vi "Autonomous Independent.vi"() -> ()   [LabVIEW 2012]
doc: "This VI is called when autonomous begins, and will automatically be terminated when autonomous ends. You can carry out timed or sensor driven robot movement independently without needing to return to the caller."
uses:
  <vilib>/Rock Robotics/WPI/Relay/WPI_RelayValue.ctl
  Robot Global Data.vi
  <vilib>/Rock Robotics/WPI/RobotDrive/WPI_RobotDriveGetSetRefNum.vi
  <vilib>/Rock Robotics/WPI/Joystick/WPI_JoystickGetSetRefNum.vi
  <vilib>/Rock Robotics/WPI/RobotDrive/WPI_RobotDriveArcadeDrive_Standard(NoSaturation).vi
panel:
  in  "Array of robot movements 2":T1(array[cluster]) {"Y Joystick Value" scale=1.0..-1.0; "X Joystick Value" scale=-1.0..1.0}
  out "Current Movement, for debugging 2":T2 {"Y Joystick Value" scale=1.0..-1.0; "X Joystick Value" scale=-1.0..1.0}
  out "Current Movement, for debugging":T2 {"Y Joystick Value" scale=1.0..-1.0; "X Joystick Value" scale=-1.0..1.0}
  in  "Array of robot movements":T1(array[cluster]) {"Y Joystick Value" scale=1.0..-1.0; "X Joystick Value" scale=-1.0..1.0}
  # "Be sure to right-click and choose Data Operations>>Make Current Value default if you want to save the array values with the VI"
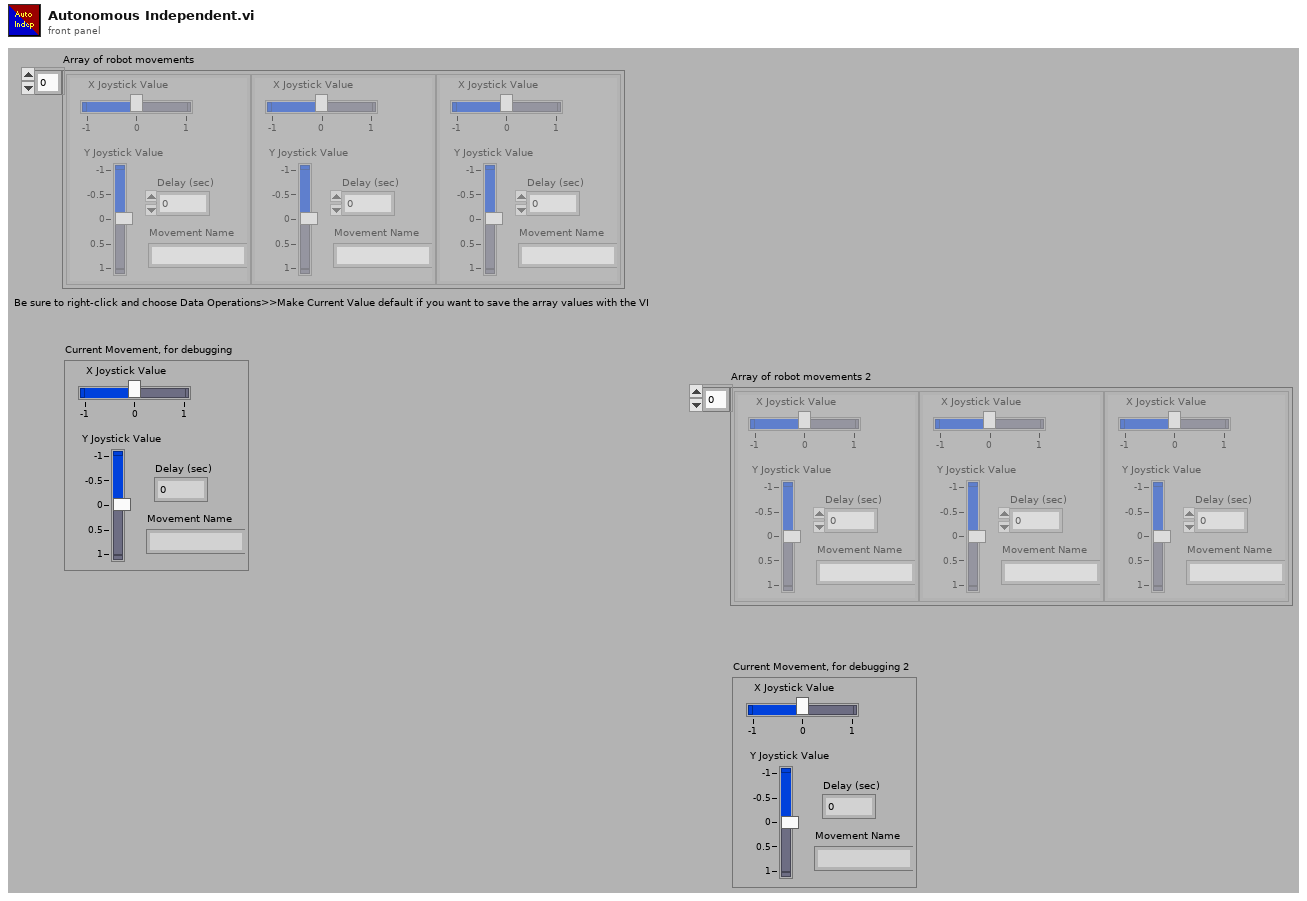
[diagram p1: front panel]
types:
  T1 = cluster{"X Joystick Value":dbl, "Y Joystick Value":dbl, "Delay (sec)":dbl, "Movement Name":string}[]
  T2 = cluster{"X Joystick Value":dbl, "Y Joystick Value":dbl, "Delay (sec)":dbl, "Movement Name":string}
  T3 = typedef "WPI_RelayValue.ctl" = enum16{"Off", "On", "Forward", "Reverse"}
  T4 = typedef "WPI_RobotDriveDevRef.ctl" = cluster{"DevStatus":errorcluster, "Motors[]":T5[], "Square Inputs":bool, "Max Output":dbl, "Isochronous":bool}
  T5 = typedef "WPI_MotorControlDeviceRef.ctl" = cluster{"DeviceStatus":errorcluster, "Type":enum16{"PWM", "CAN"}, "PWM":cluster{"Digital Module":T6, "PWM Channel":T7, "DeadBand":T8}, "CAN":cluster{"Device Number":u8, "Control Mode":T9, "Semaphore":T10, "Max Vout":dbl}, "Invert":bool, "TransformRef":T11, "InvTransformRef":T11}
  T6 = typedef "FPGA_TypedefDigitalModule.ctl" = enum16{"Digital Module 1", "Digital Module 2"}
  T7 = typedef "FPGA_DIOPWMChannel.ctl" = enum8{"PWM 1", "PWM 2", "PWM 3", "PWM 4", "PWM 5", "PWM 6", "PWM 7", "PWM 8", "PWM 9", "PWM 10", "Invalid"}
  T8 = typedef "WPI_PWMDeadband.ctl" = cluster{"Name":string, "maxPositivePwm":i32, "minPositivePwm":i32, "centerPwm":i32, "maxNegativePwm":i32, "minNegativePwm":i32, "angularRange":u16}
  T9 = typedef "WPI_CANJaguar_ControlMode.ctl" = enum8{"Percent VBus", "Current", "Speed", "Position", "Voltage"}
  T10 = typedef "Semaphore RefNum" = refnum<k1>
  T11 = typedef "WPI_PWMTransform_ConPane.ctl" = refnum<vi>
  T12 = typedef "WPI_RelayDevRef.ctl" = cluster{"DevStatus":errorcluster, "Relay Channel":T13, "Digital Module":T6, "Relay Direction":T14}
  T13 = typedef "FPGA_DIORelayChannel.ctl" = enum8{"Relay 1", "Relay 2", "Relay 3", "Relay 4", "Relay 5", "Relay 6", "Relay 7", "Relay 8", "Invalid"}
  T14 = typedef "WPI_RelayDirection.ctl" = enum16{"Both directions", "Forward only", "Reverse only"}
  T15 = typedef "WPI_JoystickDevRef.ctl" = cluster{"Device":T16}
  T16 = typedef "WPI_JoystickDeviceEnum.ctl" = enum16{"USB 1", "USB 2", "USB 3", "USB 4", "Kinect 1", "Kinect 2"}
  T17 = cluster{"axis 1 (x)":dbl, "axis 2 (y)":dbl, "axis 3 (throttle)":dbl, "axis 4":dbl, "axis 5":dbl, "axis 6":dbl}
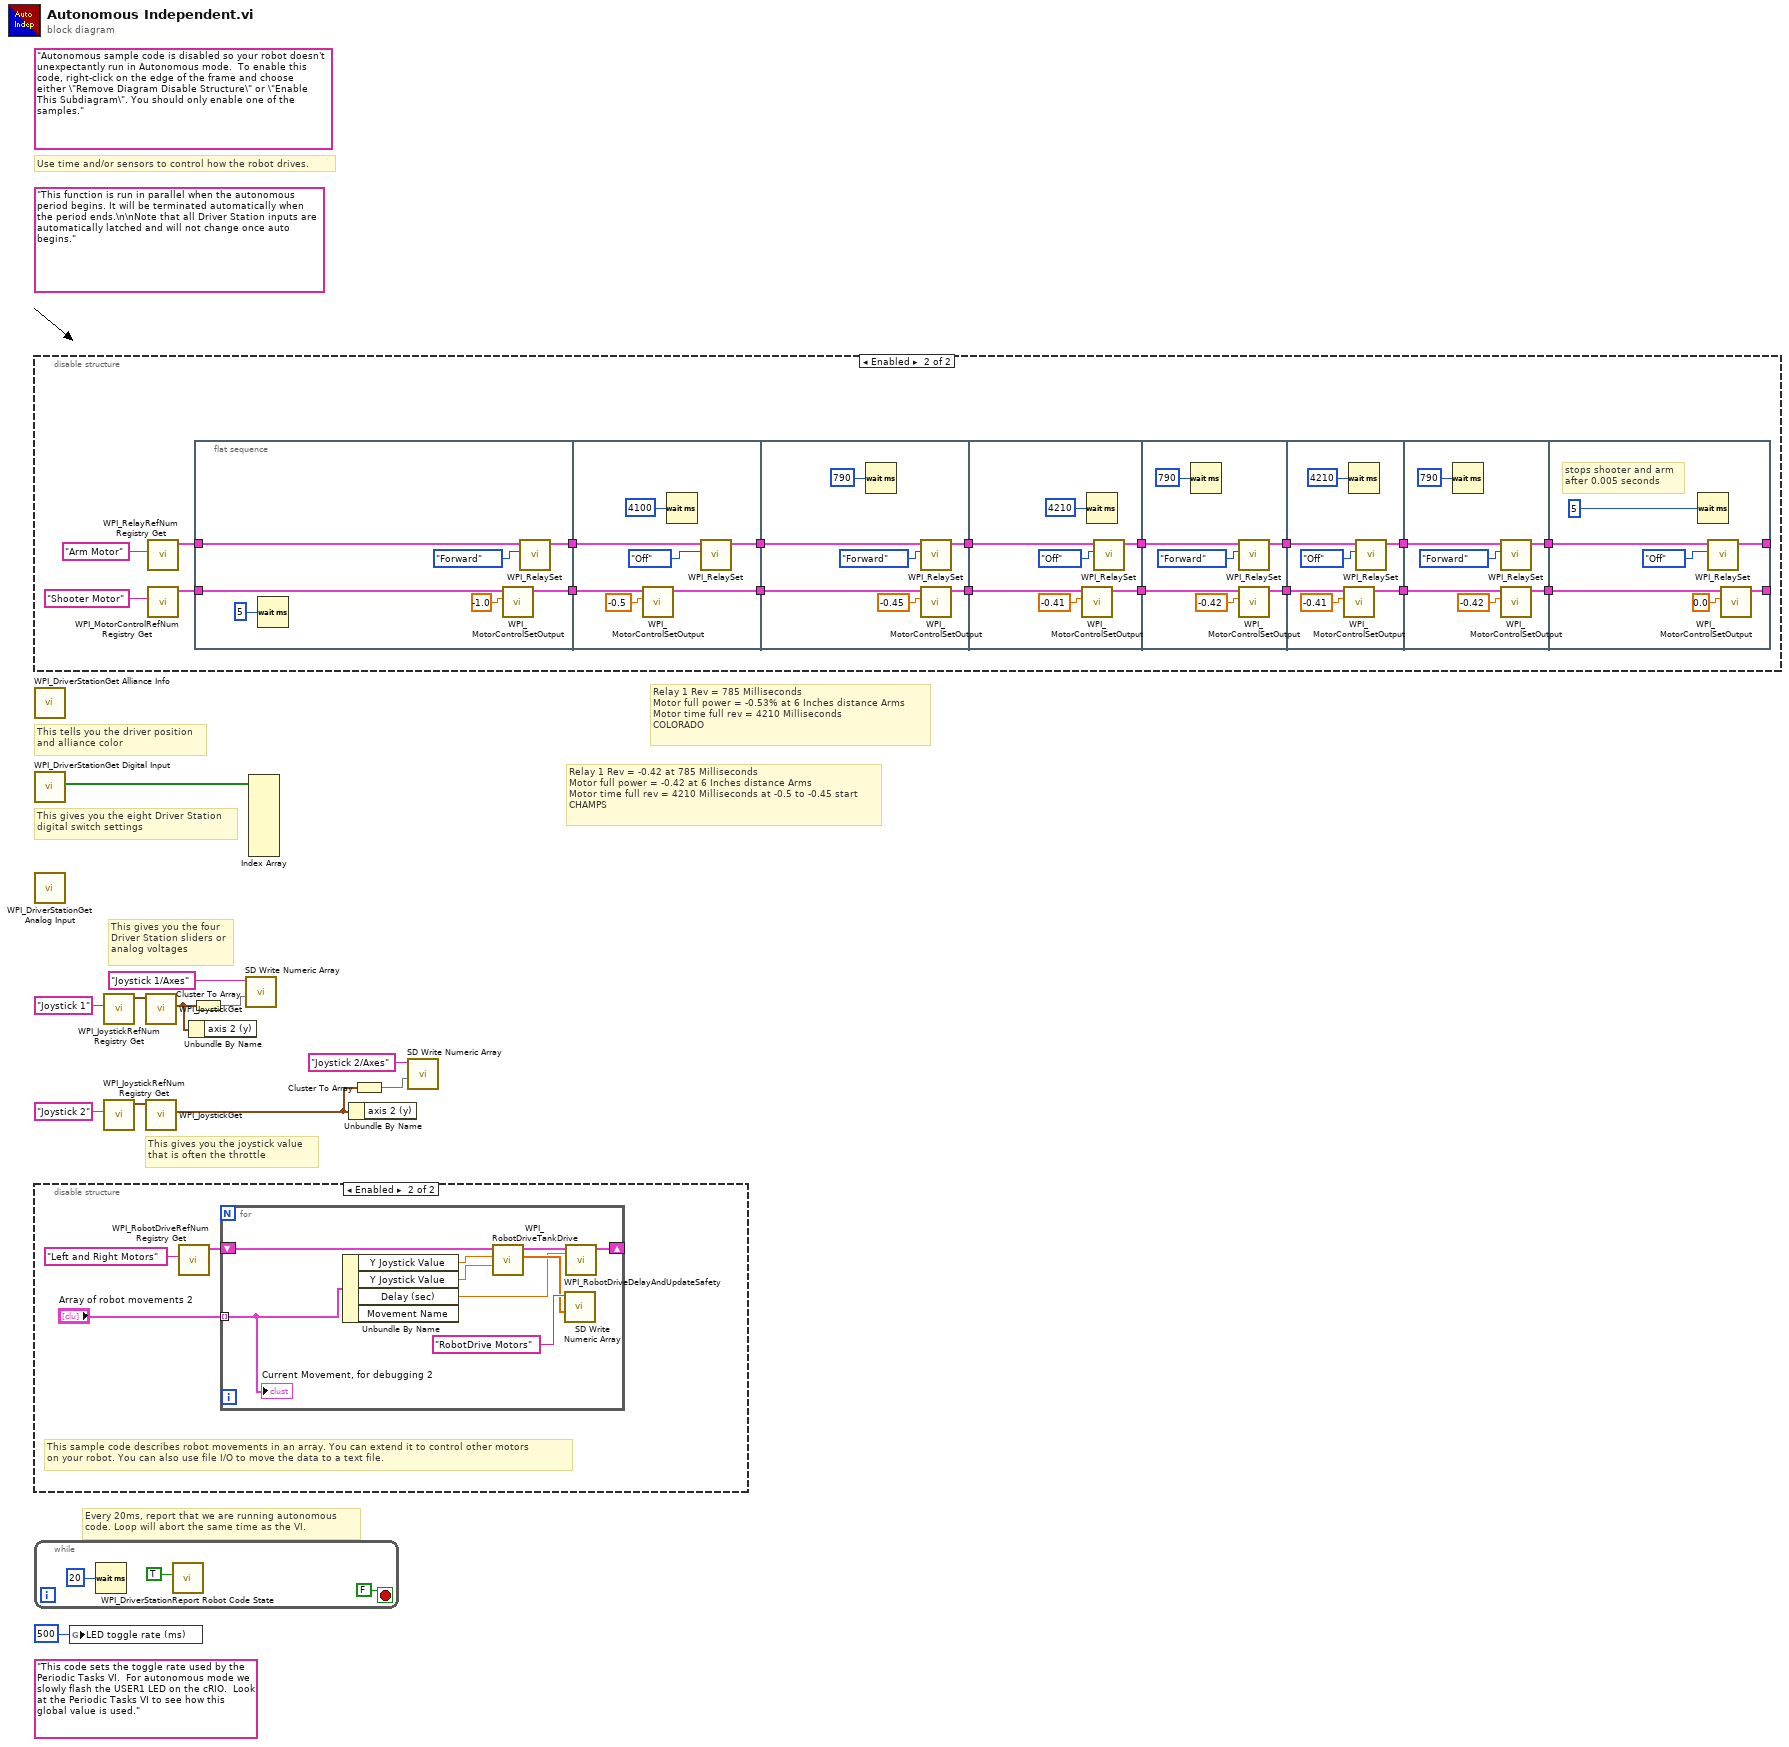
[diagram p0: block diagram]
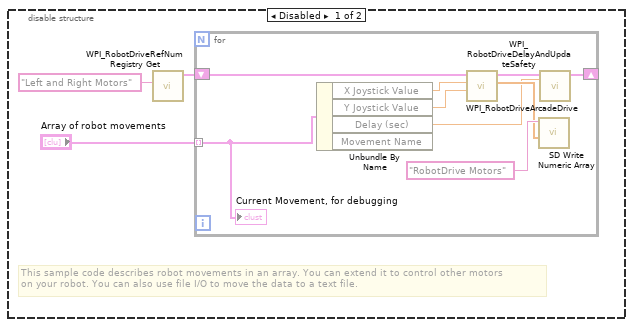
[diagram p2: hidden frame]
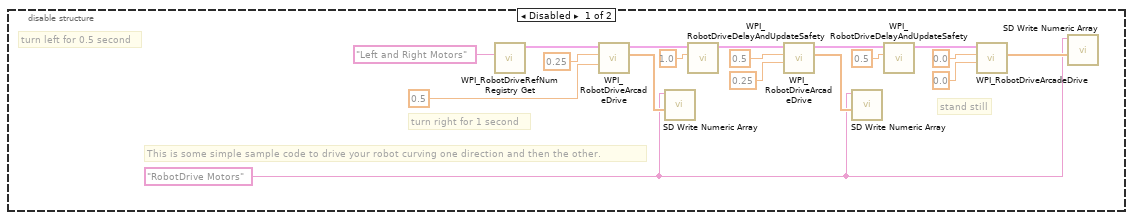
[diagram p3: hidden frame]
diagram:
  (unwired) "This code sets the toggle rate used by the Periodic Tasks VI.  For autonomous mode we slowly flash the USER1 LED on the cRIO.  Look at the Periodic Tasks VI to see how this global value is used."
  (unwired) "Autonomous sample code is disabled so your robot doesn't unexpectantly run in Autonomous mode.  To enable this code, right-click on the edge of the frame and choose either \"Remove Diagram Disable Structure\" or \"Enable This Subdiagram\". You should only enable one of the samples."
  (unwired) "This function is run in parallel when the autonomous period begins. It will be terminated automatically when the period ends.\n\nNote that all Driver Station inputs are automatically latched and will not change once auto begins."
  # "Relay 1 Rev = 785 Milliseconds\nMotor full power = -0.53% at 6 Inches distance Arms\nMotor time full rev = 4210 Milliseconds\nCOLORADO"
  # "Relay 1 Rev = -0.42 at 785 Milliseconds\nMotor full power = -0.42 at 6 Inches distance Arms\nMotor time full rev = 4210 Milliseconds at -0.5 to -0.45 start\nCHAMPS"
  # "Every 20ms, report that we are running autonomous\ncode. Loop will abort the same time as the VI."
  # "This gives you the joystick value\nthat is often the throttle"
  # "Use time and/or sensors to control how the robot drives."
  # "This tells you the driver position\nand alliance color"
  # "This gives you the eight Driver Station\ndigital switch settings"
  # "This gives you the four\nDriver Station sliders or\nanalog voltages"
  n1 = disable-structure shown="Enabled" {
    frame Disabled {
      w13 = "RobotDrive Motors" ("Name")
      # "This is some simple sample code to drive your robot curving one direction and then the other."
      # "stand still"
      # "turn left for 0.5 second"
      # "turn right for 1 second"
      n2 = call <vilib>:"WPI_RobotDriveRefNum Registry Get.vi"("refnum name"="Left and Right Motors") -> ("RobotDriveDevRef"=w17:T4)  [unwired: 1 in, 9 out]
      n3 = call-poly <vilib>:"WPI_RobotDriveArcadeDrive.vi"("Y axis value"=0.5 ("X axis value"), "X axis value"=0.25, "RobotDriveDevRef"=w17) -> ("Motor Values"=w16:dbl[], "RobotDriveDevRef"=w24:T4)  [unwired: 1 in, 6 out]
      n4 = call <vilib>:"SD Write Numeric Array.vi"("Numeric Array"=w16, "Name"=w13) -> ()  [unwired: 8 in, 2 out]
      n5 = call <vilib>:"WPI_RobotDriveDelayAndUpdateSafety.vi"("Delay (s)"=1.0, "RobotDriveDevRef"=w24) -> ("RobotDriveDevRef 2"=w23:T4)  [unwired: 8 in, 1 out]
      n6 = call-poly <vilib>:"WPI_RobotDriveArcadeDrive.vi"("Y axis value"=0.25 ("X axis value"), "X axis value"=0.5, "RobotDriveDevRef"=w23) -> ("Motor Values"=w15:dbl[], "RobotDriveDevRef"=w22:T4)  [unwired: 1 in, 6 out]
      n7 = call <vilib>:"SD Write Numeric Array.vi"("Numeric Array"=w15, "Name"=w13) -> ()  [unwired: 8 in, 2 out]
      n8 = call <vilib>:"WPI_RobotDriveDelayAndUpdateSafety.vi"("Delay (s)"=0.5, "RobotDriveDevRef"=w22) -> ("RobotDriveDevRef 2"=w21:T4)  [unwired: 8 in, 1 out]
      n9 = call-poly <vilib>:"WPI_RobotDriveArcadeDrive.vi"("Y axis value"=0.0 ("X axis value"), "X axis value"=0.0, "RobotDriveDevRef"=w21) -> ("Motor Values"=w14:dbl[])  [unwired: 1 in, 7 out]
      n10 = call <vilib>:"SD Write Numeric Array.vi"("Numeric Array"=w14, "Name"=w13) -> ()  [unwired: 8 in, 2 out]
    }
    frame Enabled {
      n11 = call <vilib>:"WPI_RelayRefNum Registry Get.vi"("refnum name"="Arm Motor") -> ("RelayDevRef"=w45:T12)  [unwired: 9 in, 1 out]
      n12 = call <vilib>:"WPI_MotorControlRefNum Registry Get.vi"("refnum name"="Shooter Motor") -> ("MotorControlDevRef"=w47:T5)  [unwired: 9 in, 1 out]
      n13 = flat-sequence {
        tunnel: w45 -> [w52]
        tunnel: w47 -> [w50]
        tunnel: [w53] -> w32
        tunnel: [w51] -> w31
        tunnel: [w60] -> w42
        tunnel: [w57] -> w41
        tunnel: w32 -> [w58]
        tunnel: w31 -> [w61]
        tunnel: w42 -> [w66]
        tunnel: w41 -> [w64]
        tunnel: [w63] -> w39
        tunnel: [w67] -> w38
        tunnel: [w74] -> w40
        tunnel: w39 -> [w72]
        tunnel: w38 -> [w75]
        tunnel: [w71] -> w37
        tunnel: [w81] -> w44
        tunnel: w40 -> [w78]
        tunnel: [w77] -> w43
        tunnel: w37 -> [w82]
        tunnel: w44 -> [w87]
        tunnel: [w88] -> w36
        tunnel: [w84] -> w34
        tunnel: w43 -> [w85]
        tunnel: w36 -> [w94]
        tunnel: [w93] -> w35
        tunnel: w34 -> [w92]
        tunnel: [w91] -> w33
        tunnel: [w102] -> _
        tunnel: [w99] -> _
        tunnel: w35 -> [w101]
        tunnel: w33 -> [w98]
        frame #0 {
          n14 = Wait (ms)(milliseconds to wait=u32 5) -> ()  [unwired: 1 out]
          n15 = call <vilib>:"WPI_MotorControlSetOutput.vi"("Output"=-1.0 ("X axis value"), "MotorControlDevRef"=w50) -> ("MotorControlDevRef"=w51:T5)  [unwired: 7 in, 2 out]
          n16 = call <vilib>:"WPI_RelaySet.vi"("RelayValue"=WPI_RelayValue."Forward", "RelayDevRef"=w52) -> ("RelayDevRef"=w53:T12)  [unwired: 8 in, 1 out]
        }
        frame #1 {
          n17 = call <vilib>:"WPI_MotorControlSetOutput.vi"("Output"=-0.5 ("X axis value"), "MotorControlDevRef"=w61) -> ("MotorControlDevRef"=w60:T5)  [unwired: 7 in, 2 out]
          n18 = Wait (ms)(milliseconds to wait=u32 4100) -> ()  [unwired: 1 out]
          n19 = call <vilib>:"WPI_RelaySet.vi"("RelayValue"=WPI_RelayValue."Off", "RelayDevRef"=w58) -> ("RelayDevRef"=w57:T12)  [unwired: 8 in, 1 out]
        }
        frame #2 {
          n20 = Wait (ms)(milliseconds to wait=u32 790) -> ()  [unwired: 1 out]
          n21 = call <vilib>:"WPI_RelaySet.vi"("RelayValue"=WPI_RelayValue."Forward", "RelayDevRef"=w64) -> ("RelayDevRef"=w63:T12)  [unwired: 8 in, 1 out]
          n22 = call <vilib>:"WPI_MotorControlSetOutput.vi"("Output"=-0.45 ("X axis value"), "MotorControlDevRef"=w66) -> ("MotorControlDevRef"=w67:T5)  [unwired: 7 in, 2 out]
        }
        frame #3 {
          n23 = call <vilib>:"WPI_MotorControlSetOutput.vi"("Output"=-0.41 ("X axis value"), "MotorControlDevRef"=w75) -> ("MotorControlDevRef"=w74:T5)  [unwired: 7 in, 2 out]
          n24 = Wait (ms)(milliseconds to wait=u32 4210) -> ()  [unwired: 1 out]
          n25 = call <vilib>:"WPI_RelaySet.vi"("RelayValue"=WPI_RelayValue."Off", "RelayDevRef"=w72) -> ("RelayDevRef"=w71:T12)  [unwired: 8 in, 1 out]
        }
        frame #4 {
          n26 = Wait (ms)(milliseconds to wait=u32 790) -> ()  [unwired: 1 out]
          n27 = call <vilib>:"WPI_RelaySet.vi"("RelayValue"=WPI_RelayValue."Forward", "RelayDevRef"=w82) -> ("RelayDevRef"=w81:T12)  [unwired: 8 in, 1 out]
          n28 = call <vilib>:"WPI_MotorControlSetOutput.vi"("Output"=-0.42 ("X axis value"), "MotorControlDevRef"=w78) -> ("MotorControlDevRef"=w77:T5)  [unwired: 7 in, 2 out]
        }
        frame #5 {
          n29 = call <vilib>:"WPI_MotorControlSetOutput.vi"("Output"=-0.41 ("X axis value"), "MotorControlDevRef"=w85) -> ("MotorControlDevRef"=w84:T5)  [unwired: 7 in, 2 out]
          n30 = Wait (ms)(milliseconds to wait=u32 4210) -> ()  [unwired: 1 out]
          n31 = call <vilib>:"WPI_RelaySet.vi"("RelayValue"=WPI_RelayValue."Off", "RelayDevRef"=w87) -> ("RelayDevRef"=w88:T12)  [unwired: 8 in, 1 out]
        }
        frame #6 {
          n32 = Wait (ms)(milliseconds to wait=u32 790) -> ()  [unwired: 1 out]
          n33 = call <vilib>:"WPI_RelaySet.vi"("RelayValue"=WPI_RelayValue."Forward", "RelayDevRef"=w94) -> ("RelayDevRef"=w93:T12)  [unwired: 8 in, 1 out]
          n34 = call <vilib>:"WPI_MotorControlSetOutput.vi"("Output"=-0.42 ("X axis value"), "MotorControlDevRef"=w92) -> ("MotorControlDevRef"=w91:T5)  [unwired: 7 in, 2 out]
        }
        frame #7 {
          # "stops shooter and arm\nafter 0.005 seconds"
          n35 = Wait (ms)(milliseconds to wait=u32 5) -> ()  [unwired: 1 out]
          n36 = call <vilib>:"WPI_RelaySet.vi"("RelayValue"=WPI_RelayValue."Off", "RelayDevRef"=w101) -> ("RelayDevRef"=w99:T12)  [unwired: 8 in, 1 out]
          n37 = call <vilib>:"WPI_MotorControlSetOutput.vi"("Output"=0.0 ("X axis value"), "MotorControlDevRef"=w98) -> ("MotorControlDevRef"=w102:T5)  [unwired: 7 in, 2 out]
        }
      }
    }
  }
  n38 = call <vilib>:"WPI_DriverStationGet Alliance Info.vi"() -> ()  [unwired: 12 out]
  n39 = call <vilib>:"WPI_DriverStationGet Digital Input.vi"() -> ("Driver Station Digital Input (1-8)"=w12:bool[])  [unwired: 11 out]
  n40 = call <vilib>:"WPI_DriverStationGet Analog Input.vi"() -> ()  [unwired: 12 out]
  n41 = disable-structure shown="Enabled" {
    frame Disabled {
      # "This sample code describes robot movements in an array. You can extend it to control other motors\non your robot. You can also use file I/O to move the data to a text file."
      n42 = call <vilib>:"WPI_RobotDriveRefNum Registry Get.vi"("refnum name"="Left and Right Motors") -> ("RobotDriveDevRef"=w106:T4)  [unwired: 1 in, 9 out]
      n43 = for {
        shift-right: [w112] -> _
        shift-left: w106 -> [w113]
        tunnel: "Array of robot movements" -> [w108] mode=indexing
        n44 = Unbundle By Name(w108) -> ("X Joystick Value"=w111:dbl, "Y Joystick Value"=w110:dbl, "Delay (sec)"=w109:dbl)  [unwired: 1 out]
        n45 = call-poly <vilib>:"WPI_RobotDriveArcadeDrive.vi"("Y axis value"=w110, "X axis value"=w111, "RobotDriveDevRef"=w113) -> ("Motor Values"=w115:dbl[], "RobotDriveDevRef"=w114:T4)  [unwired: 1 in, 6 out]
        n46 = call <vilib>:"SD Write Numeric Array.vi"("Numeric Array"=w115, "Name"="RobotDrive Motors") -> ()  [unwired: 8 in, 2 out]
        n47 = call <vilib>:"WPI_RobotDriveDelayAndUpdateSafety.vi"("Delay (s)"=w109, "RobotDriveDevRef"=w114) -> ("RobotDriveDevRef 2"=w112:T4)  [unwired: 8 in, 1 out]
        "Current Movement, for debugging" <- w108
      }
    }
    frame Enabled {
      # "This sample code describes robot movements in an array. You can extend it to control other motors\non your robot. You can also use file I/O to move the data to a text file."
      n48 = call <vilib>:"WPI_RobotDriveRefNum Registry Get.vi"("refnum name"="Left and Right Motors") -> ("RobotDriveDevRef"=w118:T4)  [unwired: 1 in, 9 out]
      n49 = for {
        shift-right: [w124] -> _
        shift-left: w118 -> [w125]
        tunnel: "Array of robot movements 2" -> [w120] mode=indexing
        n50 = Unbundle By Name(w120) -> ("Y Joystick Value"=w123:dbl, "Y Joystick Value"=w122:dbl, "Delay (sec)"=w121:dbl)  [unwired: 1 out]
        n51 = call <vilib>:"WPI_RobotDriveTankDrive.vi"("Right axis value"=w122, "Left axis value"=w123, "RobotDriveDevRef"=w125) -> ("Motor Values"=w127:dbl[], "RobotDriveDevRef"=w126:T4)  [unwired: 6 in, 1 out]
        n52 = call <vilib>:"SD Write Numeric Array.vi"("Numeric Array"=w127, "Name"="RobotDrive Motors") -> ()  [unwired: 8 in, 2 out]
        n53 = call <vilib>:"WPI_RobotDriveDelayAndUpdateSafety.vi"("Delay (s)"=w121, "RobotDriveDevRef"=w126) -> ("RobotDriveDevRef 2"=w124:T4)  [unwired: 8 in, 1 out]
        "Current Movement, for debugging 2" <- w120
      }
    }
  }
  n54 = while {
    stop <- FALSE stop-if-true
    n55 = Wait (ms)(milliseconds to wait=u32 20) -> ()  [unwired: 1 out]
    n56 = call <vilib>:"WPI_DriverStationReport Robot Code State.vi"("Autonomous"=TRUE) -> ()  [unwired: 10 in, 1 out]
  }
  n57 = global write "Robot Global Data.vi" "LED toggle rate (ms)"(u32 500 ("LED ms toggle rate")) -> ()
  n58 = call <vilib>:"WPI_JoystickRefNum Registry Get.vi"("refnum name"="Joystick 1") -> ("JoystickDevRef"=w10:T15)  [unwired: 1 in, 9 out]
  n59 = call <vilib>:"WPI_JoystickRefNum Registry Get.vi"("refnum name"="Joystick 2") -> ("JoystickDevRef"=w4:T15)  [unwired: 1 in, 9 out]
  n60 = call <vilib>:"WPI_JoystickGet.vi"("JoystickDevRef"=w10) -> ("Axes"=w7:T17)  [unwired: 1 in, 5 out]
  n61 = call <vilib>:"WPI_JoystickGet.vi"("JoystickDevRef"=w4) -> ("Axes"=w2:T17)  [unwired: 1 in, 5 out]
  n62 = Unbundle By Name(w7) -> ()  [unwired: 1 out]
  n63 = Cluster To Array(cluster=w7) -> (array=w8:dbl[])
  n64 = call <vilib>:"SD Write Numeric Array.vi"("Numeric Array"=w8, "Name"="Joystick 1/Axes") -> ()  [unwired: 8 in, 2 out]
  n65 = Index Array(array=w12) -> ()  [unwired: 8 in, 8 out]
  n66 = Unbundle By Name(w2) -> ()  [unwired: 1 out]
  n67 = Cluster To Array(cluster=w2) -> (array=w3:dbl[])
  n68 = call <vilib>:"SD Write Numeric Array.vi"("Numeric Array"=w3, "Name"="Joystick 2/Axes") -> ()  [unwired: 8 in, 2 out]
